vi "_FPGA_DDS_CycleAccumulator_v3.vi"(4 "Cycle_Increment*2^48":u64) -> (16 "Cross Quadrant?":bool, 17 "Quadrant":fxp<+,2,2>, 18 "Cross Zero Phase?":bool, 19 "RFCycleOut":u64)   [LabVIEW 2018]
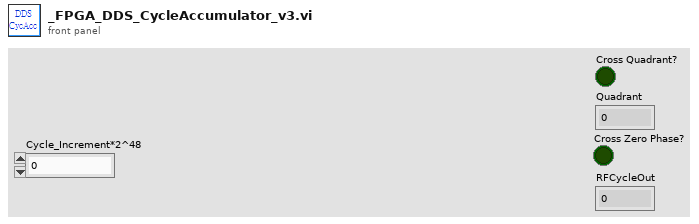
[diagram p1: front panel]
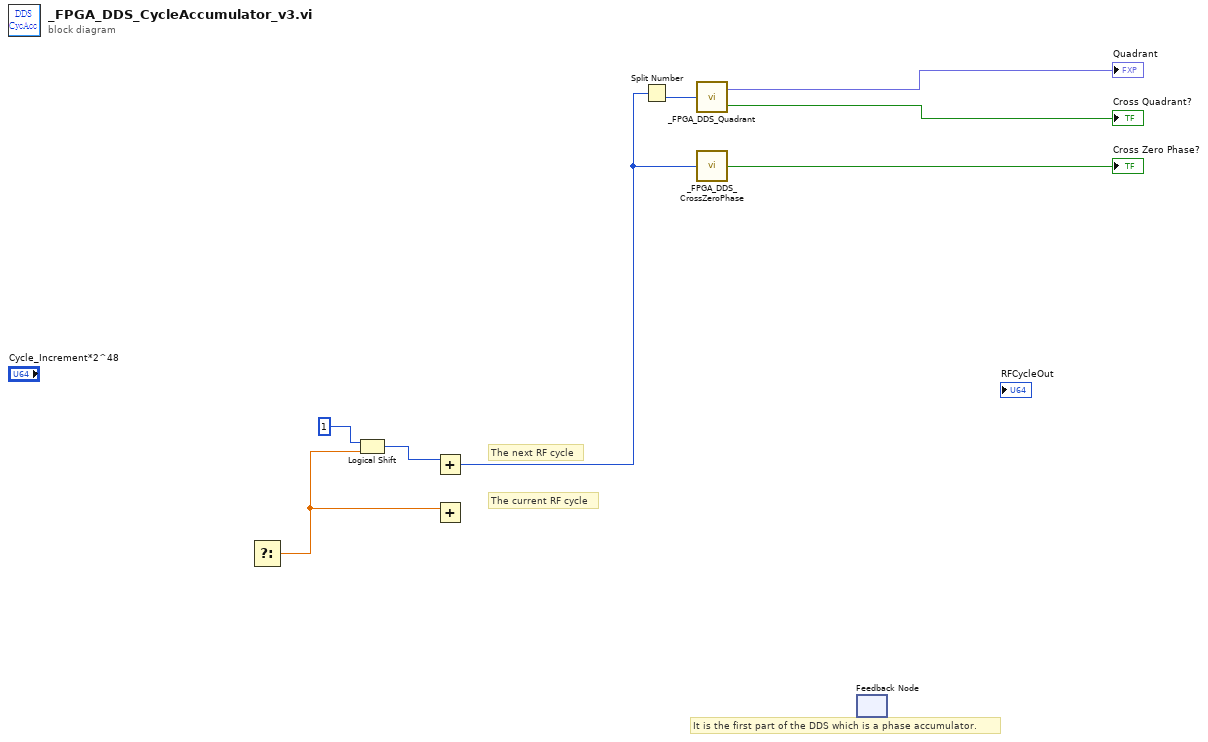
[diagram p0: block diagram]
diagram:
  # "It is the first part of the DDS which is a phase accumulator."
  # "The current RF cycle"
  # "The next RF cycle"
  n1 = Select() -> (s? t:f=w7:dbl)  [unwired: 3 in]
  n2 = Logical Shift(y=i16 1 ("n"), x=w7) -> (x << y=w6:u32)
  n3 = Add(x=w6) -> (x+y=w5:u64)  [unwired: 1 in]
  n4 = Add(x=w7) -> ()  [unwired: 1 in, 1 out]
  n5 = Split Number(x=w5) -> (lo(x)=w1:u32)  [unwired: 1 out]
  n6 = call "_FPGA_DDS_Quadrant.vi"("RfCyc_in"=w1) -> ("Cross?"=→"Cross Quadrant?":bool, "Quadrant"=→"Quadrant":fxp<+,2,2>)  [unwired: 2 in]
  n7 = call "_FPGA_DDS_CrossZeroPhase.vi"("RfCyc_in"=w5) -> ("Cross Zero Phase?"=→"Cross Zero Phase?":bool)
  n8 = feedback-in #1() -> ()  [unwired: 1 out]
  n9 = feedback #1() -> ()  [unwired: 2 in]
